vi "getConfiguration_name.vi"(8 "error in (no error)":errorcluster, 11 "OutputConfiguration.lvclass in":refnum<class "OutputConfiguration.lvclass">) -> (0 "error out":errorcluster, 2 "configuration_name":string, 3 "OutputConfiguration.lvclass out":refnum<class "OutputConfiguration.lvclass">)   [LabVIEW 2011, in "Tools.lvlib" / "DatabaseHelpers.lvlib" / "OutputConfiguration.lvclass"]
uses:
  OutputConfiguration.lvclass
  OutputConfiguration.lvclass/OutputConfiguration.ctl
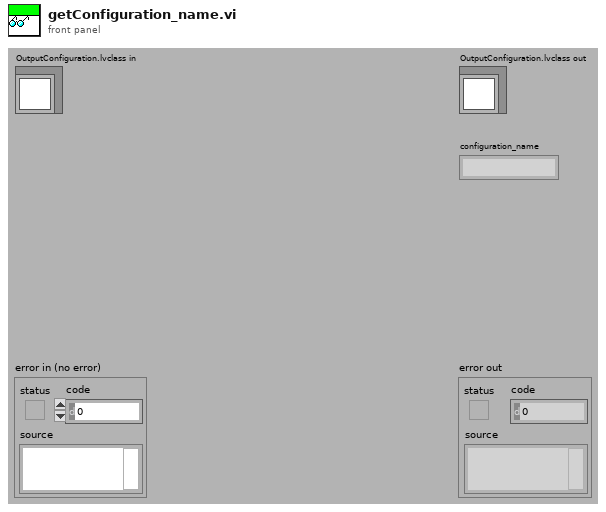
[diagram p1: front panel]
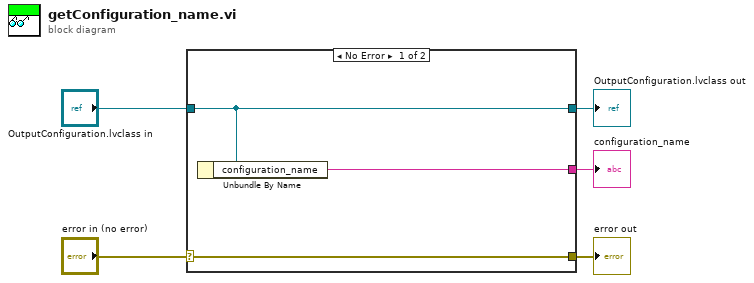
[diagram p0: block diagram]
diagram:
  n1 = case shown="No Error" "error in (no error)" {
    selector: "error in (no error)" -> [w8 w9]
    tunnel: [w8 w9] -> w4
    tunnel: [w7 w10] -> w2
    tunnel: "OutputConfiguration.lvclass in" -> [w7 w10]
    tunnel: [w6 _] -> w1
    frame No Error {
      n2 = Unbundle By Name(w7) -> ("configuration_name"=w6:string)
    }
    frame Error {
    }
  }
  "error out" <- w4
  "OutputConfiguration.lvclass out" <- w2
  "configuration_name" <- w1
